vi "ORS_DatafileWriteReadHeader_OCE.vi"(0 "file path":path, 1 "3D frame":i32, 2 "B_frame_rep":i32, 3 "read/write":u16(ring) items=["write", "read", "write_ver_2", "write_ver_3"], 4 "B_frame_per_trigger":i32, 5 "error in":errorcluster, 8 "Parameter Cluster v8":T1={"file version"=8, "data set dimension"=1, "description"="", "sampling_rate"=0.0, "samples_per_line"=0.0, "vert_range"=0.0, "various params"="", "image samples per line"=1800, "image height (crop)"=700, "CPI frequency per mm"=0.0, "Peak samp pos\n1mm (Michels)"=1, "n_channel"=1, "Buffer factor"=1, "Per Channel Params"=[{"AcqCursorList"=[{"Name"="", "Color"=0, "Style"=0, "Point Style"=0, "Name Visible"=FALSE, "Allow Drag"=FALSE, "Cursor Mode"=0, "Plot"=0, "Index"=0, "Position"={"X"=0.0, "Y"=0.0}, "X Scale"=0, "Y Scale"=0, "Watch Plots"=[], "Watch All Plots"=FALSE, "Plot Area"=0, "Label Offset"={"X"=0.0, "Y"=0.0}}], "RecalFringePhaseFit_Inv"=[], "RawDualBackgroundArray"=[], "RawSingleBackgroundArray"=[], "RawRecalFringeArray"=[], "RecalFringePhaseFit"=[], "SingleBackground"=[], "DualBackground"=[], "image crop start"=20, "cut_level_low"=40.0, "cut_level_high"=20.0, "Raw1mmFringeArray"=[], "img_bckg_offset"=119, "img_bckg_length"=20, "DVV"=[], "DVV_shift"=20, "disp_coef"=0.0}], "Galvo"={"x mirror"="", "y mirror"="", "trig out"="", "x mirror task"="", "y mirror task"="", "trig out task"="", "n_axis"=0, "params"={"n_lines"=512, "n_frames"=1, "force to zero"=FALSE, "Triggers_per_sweep"=0.0, "X center"=0.0, "X span"=0.0, "Y center"=0.0, "Y span"=0.0, "flyb.lines"=0, "n_triggers"=0, "mode"=0, "offset"=5.0, "galvo phase"=0, "span factor"=1.0, "Custom trig."={"n_f to c. trig"=150, "c. trig length"=8, "c. trig interval"=1024, "n_c. trig"=1}, "f_per_pos"=1, "n_dataset"=1, "flyback fr"=1}, "acq trig out"="", "acq trig out task"="", "sample array X"=[], "sample array Y"=[], "custom trig out"="Dev1/port0/line7", "custom trig out task"="", "FDML-box"="TCPIP0::10.153.218.51::23::SOCKET", "ACQ/Galvo"=enum."ADC/FDML", "acq trig out an task"="", "acq trig out an"="", "Galvo Trig input"="", "Galvo Clk input"="", "sample array Acq trig out an"=[]}, "n_bit"=enum."16bit", "timestamp"=""} {"data set dimension" items=["2D", "3D"]; "Galvo"."params"."n_dataset" min=1; "Galvo"."params"."X center" format="%^_3g"; "Galvo"."params"."X span" format="%^_3g"; "Galvo"."params"."Y center" format="%^_3g"; "Galvo"."params"."Y span" format="%^_3g"}) -> (14 "file refnum":refnum<file>, 17 "Parameter Cluster v8":T1={"file version"=6, "data set dimension"=1, "description"="", "sampling_rate"=0.0, "samples_per_line"=0.0, "vert_range"=0.0, "various params"="", "image samples per line"=1800, "image height (crop)"=700, "CPI frequency per mm"=0.0, "Peak samp pos\n1mm (Michels)"=1, "n_channel"=1, "Buffer factor"=1, "Per Channel Params"=[{"AcqCursorList"=[{"Name"="", "Color"=0, "Style"=0, "Point Style"=0, "Name Visible"=FALSE, "Allow Drag"=FALSE, "Cursor Mode"=0, "Plot"=0, "Index"=0, "Position"={"X"=0.0, "Y"=0.0}, "X Scale"=0, "Y Scale"=0, "Watch Plots"=[], "Watch All Plots"=FALSE, "Plot Area"=0, "Label Offset"={"X"=0.0, "Y"=0.0}}], "RecalFringePhaseFit_Inv"=[], "RawDualBackgroundArray"=[], "RawSingleBackgroundArray"=[], "RawRecalFringeArray"=[], "RecalFringePhaseFit"=[], "SingleBackground"=[], "DualBackground"=[], "image crop start"=20, "cut_level_low"=40.0, "cut_level_high"=20.0, "Raw1mmFringeArray"=[], "img_bckg_offset"=119, "img_bckg_length"=20, "DVV"=[], "DVV_shift"=20, "disp_coef"=0.0}], "Galvo"={"x mirror"="", "y mirror"="", "trig out"="", "x mirror task"="", "y mirror task"="", "trig out task"="", "n_axis"=0, "params"={"n_lines"=512, "n_frames"=1, "force to zero"=FALSE, "Triggers_per_sweep"=0.0, "X center"=0.0, "X span"=0.0, "Y center"=0.0, "Y span"=0.0, "flyb.lines"=0, "n_triggers"=0, "mode"=0, "offset"=5.0, "galvo phase"=0, "span factor"=1.0, "Custom trig."={"n_f to c. trig"=150, "c. trig length"=8, "c. trig interval"=1024, "n_c. trig"=1}, "f_per_pos"=1, "n_dataset"=1, "flyback fr"=1}, "acq trig out"="", "acq trig out task"="", "sample array X"=[], "sample array Y"=[], "custom trig out"="Dev1/port0/line7", "custom trig out task"="", "FDML-box"="TCPIP0::10.153.218.51::23::SOCKET", "ACQ/Galvo"=enum."ADC/FDML", "acq trig out an task"="", "acq trig out an"="", "Galvo Trig input"="", "Galvo Clk input"="", "sample array Acq trig out an"=[]}, "n_bit"=enum."16bit", "timestamp"=""} {"data set dimension" items=["2D", "3D"]; "Galvo"."params"."n_dataset" min=1; "Galvo"."params"."X center" format="%^_3g"; "Galvo"."params"."X span" format="%^_3g"; "Galvo"."params"."Y center" format="%^_3g"; "Galvo"."params"."Y span" format="%^_3g"}, 19 "error out":errorcluster)   [LabVIEW 2024]
uses:
  Types/ORS_Parameter_Cluster_v8.ctl
  Types/ORS_Per_Ch_params.ctl
  <vilib>/Utility/miscctls.llb/LVCursorListTypeDef.ctl
  Types/ORS_Galvo.ctl
  Types/ORS_Galvo_params.ctl
panel:
  out "B_frame_per_trigger 2":i32
  out "B_frame_rep 2":i32
  out "3D frame 2":i32
  out "offset 2":i32
  out "length 2":i32
  out "length":i32
  out "offset":i32
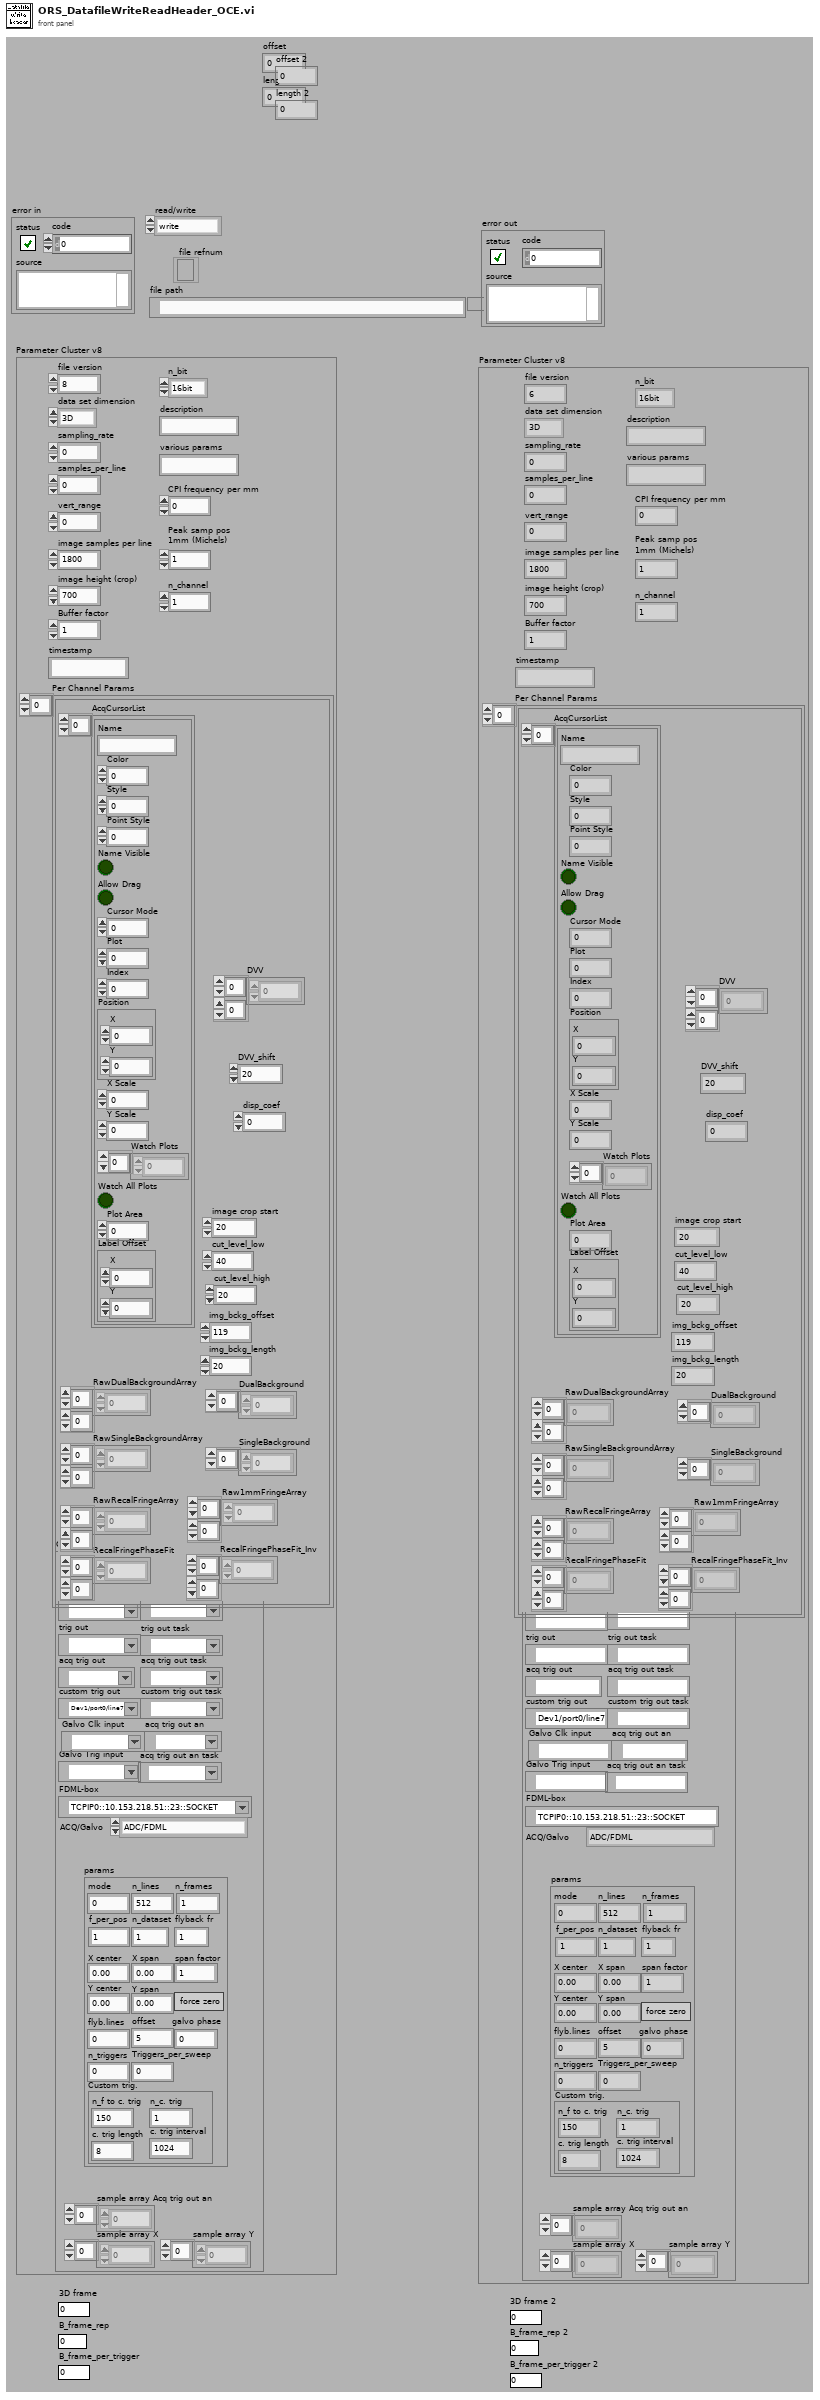
[diagram p1: front panel]
types:
  T1 = typedef "ORS_Parameter_Cluster_v8.ctl" = cluster{"file version":u32, "data set dimension":u16, "description":string, "sampling_rate":dbl, "samples_per_line":dbl, "vert_range":dbl, "various params":string, "image samples per line":i32, "image height (crop)":i32, "CPI frequency per mm":dbl, "Peak samp pos\n1mm (Michels)":i32, "n_channel":i32, "Buffer factor":i32, "Per Channel Params":T2, "Galvo":T4, "n_bit":enum16{"8bit", "16bit"}, "timestamp":string}
  T2 = typedef "ORS_Per_Ch_params.ctl" = cluster{"AcqCursorList":T3, "RecalFringePhaseFit_Inv":dbl[][], "RawDualBackgroundArray":i16[][], "RawSingleBackgroundArray":i16[][], "RawRecalFringeArray":i16[][], "RecalFringePhaseFit":dbl[][], "SingleBackground":i16[], "DualBackground":i16[], "image crop start":i32, "cut_level_low":dbl, "cut_level_high":dbl, "Raw1mmFringeArray":i16[][], "img_bckg_offset":i32, "img_bckg_length":i32, "DVV":i16[][], "DVV_shift":i32, "disp_coef":dbl}[]
  T3 = typedef "LVCursorListTypeDef.ctl" = cluster{"Name":string, "Color":u32, "Style":u8, "Point Style":u8, "Name Visible":bool, "Allow Drag":bool, "Cursor Mode":u32, "Plot":i32, "Index":i32, "Position":cluster{"X":dbl, "Y":dbl}, "X Scale":u32, "Y Scale":u32, "Watch Plots":i32[], "Watch All Plots":bool, "Plot Area":i32, "Label Offset":cluster{"X":dbl, "Y":dbl}}[]
  T4 = typedef "ORS_Galvo.ctl" = cluster{"x mirror":tag, "y mirror":tag, "trig out":tag, "x mirror task":refnum<k21>, "y mirror task":refnum<k21>, "trig out task":refnum<k21>, "n_axis":i32, "params":T5, "acq trig out":tag, "acq trig out task":refnum<k21>, "sample array X":dbl[], "sample array Y":dbl[], "custom trig out":tag, "custom trig out task":refnum<k21>, "FDML-box":refnum<visa-resource-name>, "ACQ/Galvo":enum16{"ADC/FDML", "NI_DAQ", "ADC"}, "acq trig out an task":refnum<k21>, "acq trig out an":tag, "Galvo Trig input":tag, "Galvo Clk input":tag, "sample array Acq trig out an":dbl[]}
  T5 = typedef "ORS_Galvo_params.ctl" = cluster{"n_lines":i32, "n_frames":i32, "force to zero":bool, "Triggers_per_sweep":dbl, "X center":dbl, "X span":dbl, "Y center":dbl, "Y span":dbl, "flyb.lines":i32, "n_triggers":i32, "mode":i32, "offset":dbl, "galvo phase":i32, "span factor":dbl, "Custom trig.":cluster{"n_f to c. trig":i32, "c. trig length":i32, "c. trig interval":i32, "n_c. trig":i32}, "f_per_pos":i32, "n_dataset":u32, "flyback fr":u16}
  T6 = enum16{"big-endian, network order", "native, host order", "little-endian"}
  T7 = cluster{"AcqCursorList":T3, "RecalFringePhaseFit_Inv":dbl[][], "RawDualBackgroundArray":i16[][], "RawSingleBackgroundArray":i16[][], "RawRecalFringeArray":i16[][], "RecalFringePhaseFit":dbl[][], "SingleBackground":i16[], "DualBackground":i16[], "image crop start":i32, "cut_level_low":dbl, "cut_level_high":dbl, "Raw1mmFringeArray":i16[][], "img_bckg_offset":i32, "img_bckg_length":i32, "DVV":i16[][], "DVV_shift":i32, "disp_coef":dbl}
  T8 = cluster{"Name":string, "Color":u32, "Style":u8, "Point Style":u8, "Name Visible":bool, "Allow Drag":bool, "Cursor Mode":u32, "Plot":i32, "Index":i32, "Position":cluster{"X":dbl, "Y":dbl}, "X Scale":u32, "Y Scale":u32, "Watch Plots":i32[], "Watch All Plots":bool, "Plot Area":i32, "Label Offset":cluster{"X":dbl, "Y":dbl}}
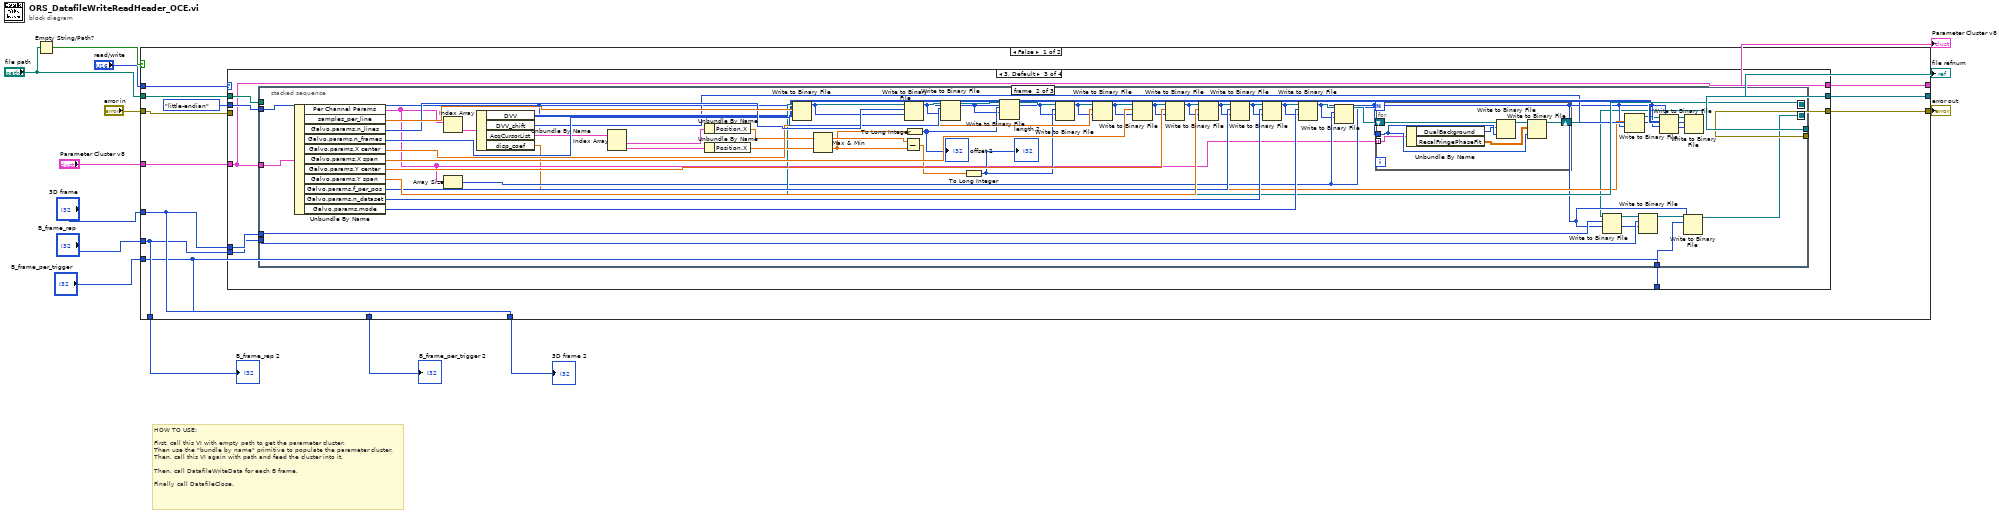
[diagram p0: block diagram]
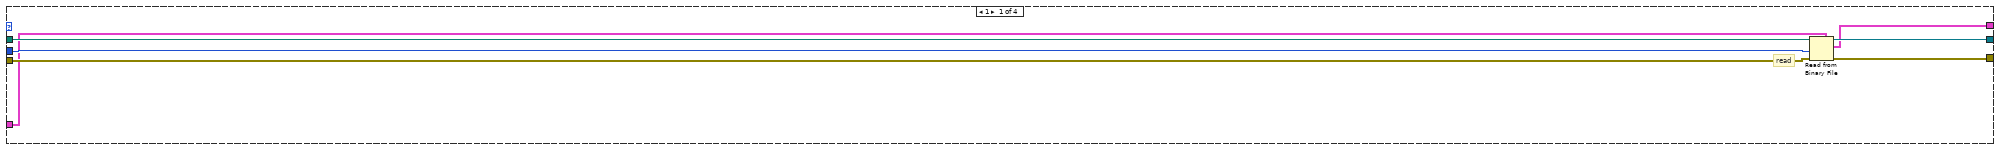
[diagram p2: hidden frame]
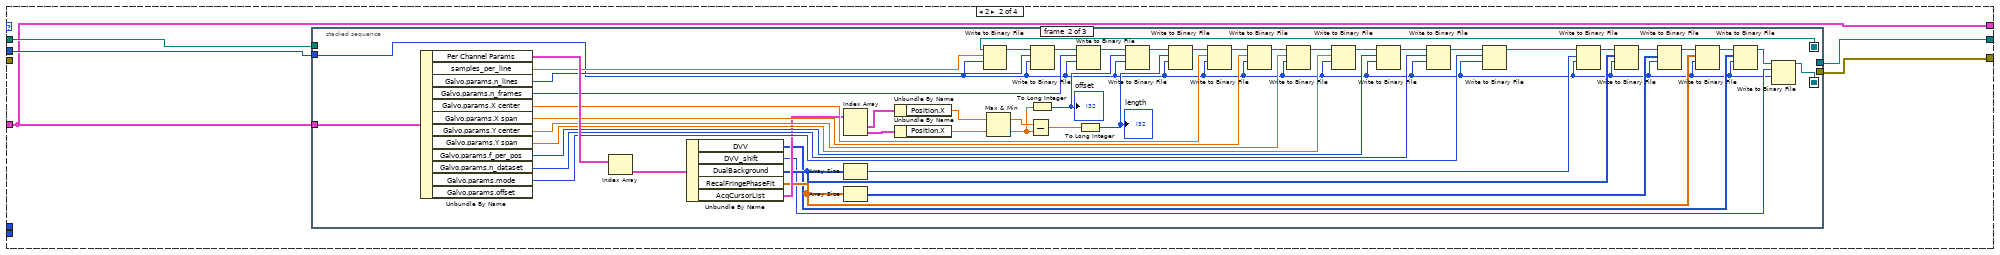
[diagram p3: hidden frame]
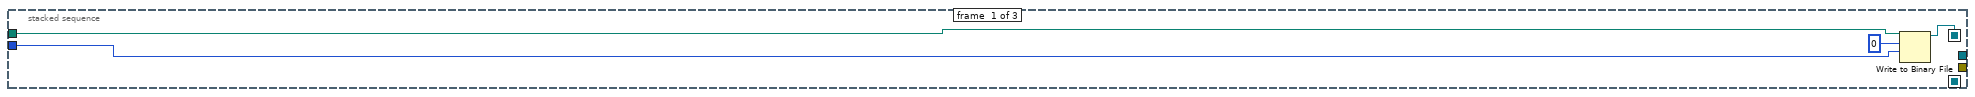
[diagram p4: hidden frame]
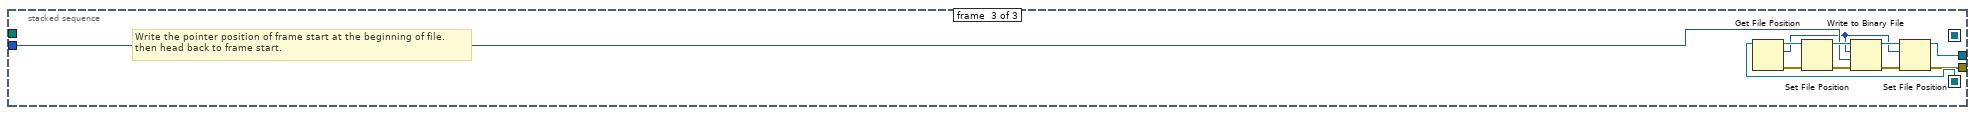
[diagram p5: hidden frame]
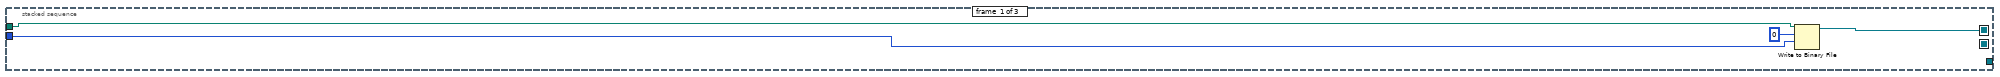
[diagram p6: hidden frame]
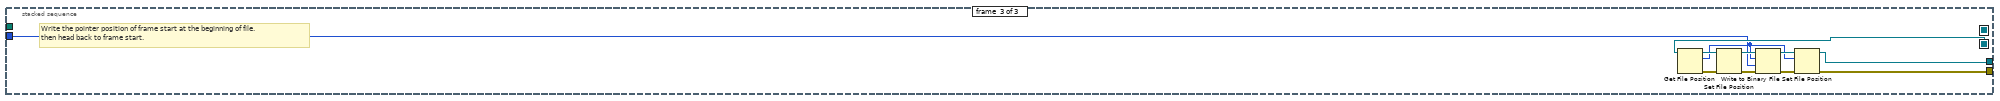
[diagram p7: hidden frame]
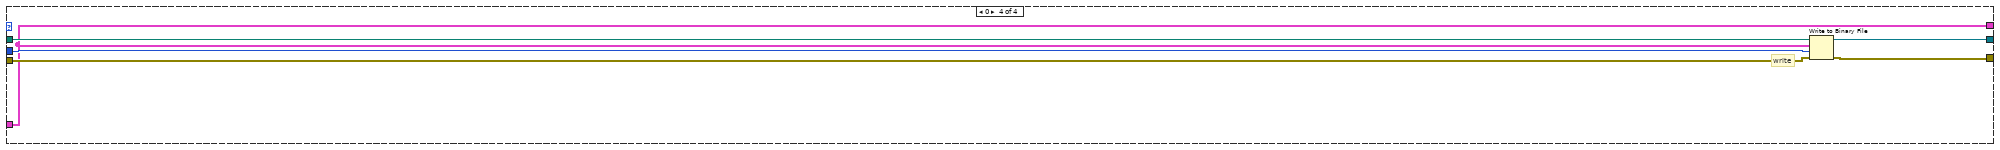
[diagram p8: hidden frame]
diagram:
  # "HOW TO USE:\n\nFirst, call this VI with empty path to get the parameter cluster. \nThen use the \"bundle by name\" primitive to populate the parameter cluster.\nThen, call this VI again with path and feed the cluster into it. \n\nThen, call DatafileWriteData for each B frame. \n\nFinally call DatafileClose."
  n1 = Empty String/Path?(string/path="file path") -> (empty?=w11:bool)
  n2 = case shown="False" w11 {
    tunnel: "error in" -> [w25 w194]
    tunnel: [w24 w194] -> w14
    tunnel: [w23 _] -> w13
    tunnel: "Parameter Cluster v8" -> [w22 w193]
    tunnel: "file path" -> [w20 _]
    tunnel: "read/write" -> [w19 _]
    tunnel: [w18 w193] -> w8
    tunnel: "3D frame" -> [w17 w192]
    tunnel: "B_frame_rep" -> [w16 w191]
    tunnel: "B_frame_per_trigger" -> [w15 w190]
    tunnel: [w17 w192] -> w3
    tunnel: [w16 w191] -> w2
    tunnel: [w15 w190] -> w1
    frame False {
      n3 = case shown="3, Default" w19 {
        tunnel: w25 -> [w32 _ _ w189]
        tunnel: [w31 w33 w105 w188] -> w24
        tunnel: [w30 w34 w106 w187] -> w23
        tunnel: w22 -> [w27 w35 w107 w184]
        tunnel: T6."little-endian" ("byte order (0:big-endian, network order)") -> [w29 w36 w108 w186]
        tunnel: w20 -> [w28 w37 w109 w185]
        tunnel: [w26 w35 w107 w184] -> w18
        tunnel: w17 -> [_ _ w104 _]
        tunnel: w16 -> [_ _ w103 _]
        tunnel: w15 -> [_ _ w102 _]
        frame 1 {
          # "read"
          n4 = Read from Binary File(5:w27, 8:w32, 9:w29, 11:w28) -> (0:w31:errorcluster, 2:w26:T1, 3:w30:refnum<file>)  [unwired: 2 in, 1 out]
        }
        frame 2 {
          n5 = stacked-sequence {
            seq-local: [_ w45 _] -> [_ _ w101]
            seq-local: [w40 _ _] -> [_ w50 _]
            tunnel: w37 -> [w41 _ _]
            tunnel: w36 -> [w39 w42 w98]
            tunnel: w35 -> [_ w52 _]
            tunnel: [_ _ w95] -> w34
            tunnel: [_ _ w91] -> w33
            frame #0 {
              n6 = Write to Binary File(file (use dialog)=w41, data=u32 0, 9:w39) -> (refnum out=w40:refnum<file>)  [unwired: 3 in, 2 out]
            }
            frame #1 {
              n7 = Unbundle By Name(w52) -> ("Per Channel Params"=w90:T2, "samples_per_line"=w88:dbl, "Galvo.params.n_lines"=w87:i32, "Galvo.params.n_frames"=w86:i32, "Galvo.params.X center"=w85:dbl, "Galvo.params.X span"=w84:dbl, "Galvo.params.Y center"=w83:dbl, "Galvo.params.Y span"=w82:dbl, "Galvo.params.f_per_pos"=w81:i32, "Galvo.params.n_dataset"=w80:u32, "Galvo.params.mode"=w79:i32)  [unwired: 1 out]
              n8 = Index Array(array=w90) -> (element=w89:T7)  [unwired: 1 in]
              n9 = Unbundle By Name(w89) -> ("DVV"=w44:i16[][], "DVV_shift"=w43:i32, "DualBackground"=w56:i16[], "RecalFringePhaseFit"=w48:dbl[][], "AcqCursorList"=w64:T3)
              n10 = Index Array(array=w64) -> (element #1=w71:T8, element #2=w70:T8)  [unwired: 2 in]
              n11 = Array Size(array=w56) -> (size(s)=w51:i32)
              n12 = Array Size(array=w48) -> (size(s)=w54:i32[])
              n13 = Unbundle By Name(w71) -> ("Position.X"=w69:dbl)
              n14 = Unbundle By Name(w70) -> ("Position.X"=w68:dbl)
              n15 = Write to Binary File(file (use dialog)=w50, data=w88, 9:w42) -> (refnum out=w49:refnum<file>)  [unwired: 3 in, 2 out]
              n16 = Max & Min(x=w69, y=w68) -> (max(x,y)=w67:dbl, min(x,y)=w65:dbl)
              n17 = Subtract(x=w67, y=w65) -> (x-y=w66:dbl)
              n18 = Write to Binary File(file (use dialog)=w49, data=w87, 9:w42) -> (refnum out=w78:refnum<file>)  [unwired: 3 in, 2 out]
              n19 = To Long Integer(number=w65) -> (32bit integer=w60:i32)
              "offset" <- w60
              n20 = Write to Binary File(file (use dialog)=w78, data=w86, 9:w42) -> (refnum out=w63:refnum<file>)  [unwired: 3 in, 2 out]
              n21 = To Long Integer(number=w66) -> (32bit integer=w59:i32)
              "length" <- w59
              n22 = Write to Binary File(file (use dialog)=w63, data=w60, 9:w42) -> (refnum out=w62:refnum<file>)  [unwired: 3 in, 2 out]
              n23 = Write to Binary File(file (use dialog)=w62, data=w59, 9:w42) -> (refnum out=w61:refnum<file>)  [unwired: 3 in, 2 out]
              n24 = Write to Binary File(file (use dialog)=w61, data=w85, 9:w42) -> (refnum out=w77:refnum<file>)  [unwired: 3 in, 2 out]
              n25 = Write to Binary File(file (use dialog)=w77, data=w84, 9:w42) -> (refnum out=w76:refnum<file>)  [unwired: 3 in, 2 out]
              n26 = Write to Binary File(file (use dialog)=w76, data=w83, 9:w42) -> (refnum out=w75:refnum<file>)  [unwired: 3 in, 2 out]
              n27 = Write to Binary File(file (use dialog)=w75, data=w82, 9:w42) -> (refnum out=w74:refnum<file>)  [unwired: 3 in, 2 out]
              n28 = Write to Binary File(file (use dialog)=w74, data=w81, 9:w42) -> (refnum out=w73:refnum<file>)  [unwired: 3 in, 2 out]
              n29 = Write to Binary File(file (use dialog)=w73, data=w80, 9:w42) -> (refnum out=w72:refnum<file>)  [unwired: 3 in, 2 out]
              n30 = Write to Binary File(file (use dialog)=w72, data=w79, 9:w42) -> (refnum out=w58:refnum<file>)  [unwired: 3 in, 2 out]
              n31 = Write to Binary File(file (use dialog)=w58, data=w51, 9:w42) -> (refnum out=w57:refnum<file>)  [unwired: 3 in, 2 out]
              n32 = Write to Binary File(file (use dialog)=w57, data=w56, 9:w42) -> (refnum out=w55:refnum<file>)  [unwired: 3 in, 2 out]
              n33 = Write to Binary File(file (use dialog)=w55, data=w54, 9:w42) -> (refnum out=w53:refnum<file>)  [unwired: 3 in, 2 out]
              n34 = Write to Binary File(file (use dialog)=w53, data=w48, 9:w42) -> (refnum out=w47:refnum<file>)  [unwired: 3 in, 2 out]
              n35 = Write to Binary File(file (use dialog)=w47, data=w44, 9:w42) -> (refnum out=w46:refnum<file>)  [unwired: 3 in, 2 out]
              n36 = Write to Binary File(file (use dialog)=w46, data=w43, 9:w42) -> (refnum out=w45:refnum<file>)  [unwired: 3 in, 2 out]
            }
            frame #2 {
              # "Write the pointer position of frame start at the beginning of file.\nthen head back to frame start."
              n37 = Get File Position(7:w101) -> (0:w94:errorcluster, 2:w96:i64, 3:w100:refnum<file>)  [unwired: 1 in]
              n38 = Set File Position(refnum=w100, error in=w94) -> (refnum out=w99:refnum<file>, error out=w93:errorcluster)  [unwired: 2 in]
              n39 = Write to Binary File(file (use dialog)=w99, data=w96, error in=w93, 9:w98) -> (refnum out=w97:refnum<file>, error out=w92:errorcluster)  [unwired: 2 in, 1 out]
              n40 = Set File Position(offset (in bytes) (0)=w96, refnum=w97, error in=w92) -> (refnum out=w95:refnum<file>, error out=w91:errorcluster)  [unwired: 1 in]
            }
          }
        }
        frame 3, Default {
          n41 = stacked-sequence {
            seq-local: [_ w114 _] -> [_ _ w183]
            seq-local: [w112 _ _] -> [_ w131 _]
            tunnel: w109 -> [w113 _ _]
            tunnel: w108 -> [w111 w118 w180]
            tunnel: w107 -> [_ w132 _]
            tunnel: [_ _ w177] -> w106
            tunnel: [_ _ w173] -> w105
            tunnel: w104 -> [_ w121 _]
            tunnel: w103 -> [_ w120 _]
            tunnel: w102 -> [_ w119 _]
            frame #0 {
              n42 = Write to Binary File(file (use dialog)=w113, data=u32 0, 9:w111) -> (refnum out=w112:refnum<file>)  [unwired: 3 in, 2 out]
            }
            frame #1 {
              n43 = Unbundle By Name(w132) -> ("Per Channel Params"=w125:T2, "samples_per_line"=w164:dbl, "Galvo.params.n_lines"=w163:i32, "Galvo.params.n_frames"=w162:i32, "Galvo.params.X center"=w161:dbl, "Galvo.params.X span"=w160:dbl, "Galvo.params.Y center"=w159:dbl, "Galvo.params.Y span"=w158:dbl, "Galvo.params.f_per_pos"=w157:i32, "Galvo.params.n_dataset"=w156:u32, "Galvo.params.mode"=w155:i32)
              n44 = Index Array(array=w125) -> (element=w165:T7)  [unwired: 1 in]
              n45 = Array Size(array=w125) -> (size(s)=w126:i32)
              n46 = Unbundle By Name(w165) -> ("DVV"=w128:i16[][], "DVV_shift"=w127:i32, "AcqCursorList"=w140:T3, "disp_coef"=w124:dbl)
              n47 = Index Array(array=w140) -> (element #1=w147:T8, element #2=w146:T8)  [unwired: 2 in]
              n48 = Unbundle By Name(w147) -> ("Position.X"=w145:dbl)
              n49 = Unbundle By Name(w146) -> ("Position.X"=w144:dbl)
              n50 = Write to Binary File(file (use dialog)=w131, data=w164, 9:w118) -> (refnum out=w130:refnum<file>)  [unwired: 3 in, 2 out]
              n51 = Max & Min(x=w145, y=w144) -> (max(x,y)=w143:dbl, min(x,y)=w141:dbl)
              n52 = Subtract(x=w143, y=w141) -> (x-y=w142:dbl)
              n53 = Write to Binary File(file (use dialog)=w130, data=w163, 9:w118) -> (refnum out=w154:refnum<file>)  [unwired: 3 in, 2 out]
              n54 = To Long Integer(number=w141) -> (32bit integer=w136:i32)
              "offset 2" <- w136
              n55 = Write to Binary File(file (use dialog)=w154, data=w162, 9:w118) -> (refnum out=w139:refnum<file>)  [unwired: 3 in, 2 out]
              n56 = To Long Integer(number=w142) -> (32bit integer=w135:i32)
              "length 2" <- w135
              n57 = Write to Binary File(file (use dialog)=w139, data=w136, 9:w118) -> (refnum out=w138:refnum<file>)  [unwired: 3 in, 2 out]
              n58 = Write to Binary File(file (use dialog)=w138, data=w135, 9:w118) -> (refnum out=w137:refnum<file>)  [unwired: 3 in, 2 out]
              n59 = Write to Binary File(file (use dialog)=w137, data=w161, 9:w118) -> (refnum out=w153:refnum<file>)  [unwired: 3 in, 2 out]
              n60 = Write to Binary File(file (use dialog)=w153, data=w160, 9:w118) -> (refnum out=w152:refnum<file>)  [unwired: 3 in, 2 out]
              n61 = Write to Binary File(file (use dialog)=w152, data=w159, 9:w118) -> (refnum out=w151:refnum<file>)  [unwired: 3 in, 2 out]
              n62 = Write to Binary File(file (use dialog)=w151, data=w158, 9:w118) -> (refnum out=w150:refnum<file>)  [unwired: 3 in, 2 out]
              n63 = Write to Binary File(file (use dialog)=w150, data=w157, 9:w118) -> (refnum out=w149:refnum<file>)  [unwired: 3 in, 2 out]
              n64 = Write to Binary File(file (use dialog)=w149, data=w156, 9:w118) -> (refnum out=w148:refnum<file>)  [unwired: 3 in, 2 out]
              n65 = Write to Binary File(file (use dialog)=w148, data=w155, 9:w118) -> (refnum out=w134:refnum<file>)  [unwired: 3 in, 2 out]
              n66 = Write to Binary File(file (use dialog)=w134, data=w126, 9:w118) -> (refnum out=w133:refnum<file>)  [unwired: 3 in, 2 out]
              n67 = for {
                N: w126 -> [_]
                tunnel: w118 -> [w170]
                shift-right: [w171] -> w116
                shift-left: w133 -> [w172]
                tunnel: w125 -> [w166] mode=indexing
                n68 = Unbundle By Name(w166) -> ("DualBackground"=w168:i16[], "RecalFringePhaseFit"=w167:dbl[][])
                n69 = Write to Binary File(file (use dialog)=w172, data=w168, 9:w170) -> (refnum out=w169:refnum<file>)  [unwired: 3 in, 2 out]
                n70 = Write to Binary File(file (use dialog)=w169, data=w167, 9:w170) -> (refnum out=w171:refnum<file>)  [unwired: 3 in, 2 out]
              }
              n71 = Write to Binary File(file (use dialog)=w116, data=w124, 9:w118) -> (refnum out=w117:refnum<file>)  [unwired: 3 in, 2 out]
              n72 = Write to Binary File(file (use dialog)=w117, data=w128, 9:w118) -> (refnum out=w129:refnum<file>)  [unwired: 3 in, 2 out]
              n73 = Write to Binary File(file (use dialog)=w129, data=w127, 9:w118) -> (refnum out=w115:refnum<file>)  [unwired: 3 in, 2 out]
              n74 = Write to Binary File(file (use dialog)=w115, data=w121, 9:w118) -> (refnum out=w123:refnum<file>)  [unwired: 3 in, 2 out]
              n75 = Write to Binary File(file (use dialog)=w123, data=w120, 9:w118) -> (refnum out=w122:refnum<file>)  [unwired: 3 in, 2 out]
              n76 = Write to Binary File(file (use dialog)=w122, data=w119, 9:w118) -> (refnum out=w114:refnum<file>)  [unwired: 3 in, 2 out]
            }
            frame #2 {
              # "Write the pointer position of frame start at the beginning of file.\nthen head back to frame start."
              n77 = Get File Position(7:w183) -> (0:w176:errorcluster, 2:w178:i64, 3:w182:refnum<file>)  [unwired: 1 in]
              n78 = Set File Position(refnum=w182, error in=w176) -> (refnum out=w181:refnum<file>, error out=w175:errorcluster)  [unwired: 2 in]
              n79 = Write to Binary File(file (use dialog)=w181, data=w178, error in=w175, 9:w180) -> (refnum out=w179:refnum<file>, error out=w174:errorcluster)  [unwired: 2 in, 1 out]
              n80 = Set File Position(offset (in bytes) (0)=w178, refnum=w179, error in=w174) -> (refnum out=w177:refnum<file>, error out=w173:errorcluster)  [unwired: 1 in]
            }
          }
        }
        frame 0 {
          # "write"
          n81 = Write to Binary File(file (use dialog)=w185, data=w184, error in=w189, 9:w186) -> (refnum out=w187:refnum<file>, error out=w188:errorcluster)  [unwired: 2 in, 1 out]
        }
      }
    }
    frame True {
    }
  }
  "error out" <- w14
  "file refnum" <- w13
  "Parameter Cluster v8" <- w8
  "3D frame 2" <- w3
  "B_frame_rep 2" <- w2
  "B_frame_per_trigger 2" <- w1
